vi "Launcher.vi"   [LabVIEW 2023, in "Example GUI View Actor.lvlib"]
uses:
  Example Controller Actor/Example Controller Actor.lvclass
  Example GUI View Actor.lvlib
  Timed Loop Controller/Timed Loop Controller/Timed Loop Controller.lvclass
  <vilib>/ActorFramework/Actor/Actor.lvclass
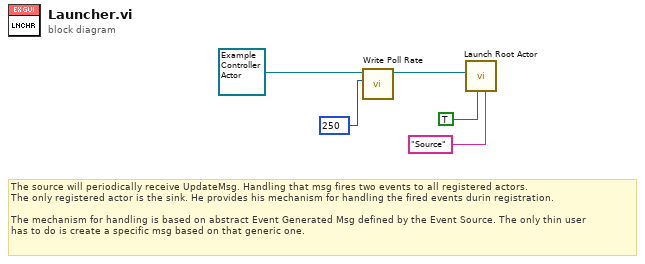
[diagram p0: block diagram]
diagram:
  # "The source will periodically receive UpdateMsg. Handling that msg fires two events to all registered actors.\nThe only registered actor is the sink. He provides his mechanism for handling the fired events durin registration.\n\nThe mechanism for handling is based on abstract Event Generated Msg defined by the Event Source. The only thin user\nhas to do is create a specific msg based on that generic one."
  n1 = call "Write Poll Rate.vi"("Poll Rate"=u32 250, "Timed Loop Controller in"=refnum<class "Example Controller Actor.lvclass"> refnum ("Example GUI View Actor.lvlib:Example Controller Actor.lvclass")) -> ("Timed Loop Controller out"=w5:refnum<class "Example Controller Actor.lvclass">)  [unwired: 8 in, 1 out]
  n2 = call <vilib>:"Launch Root Actor.vi"("Debug Alias"="Source", "Open Actor Core front panel? (F)"=TRUE, "Actor"=w5) -> ()  [unwired: 7 in, 2 out]
